vi "TrapezoidalMotionProfile.vi"(6 "Initialize":bool, 7 "dt":dbl=0.02 format="%#_13g", 10 "Time":dbl, 11 "Config":T2={"TargetPos"=10.0, "InitalPos"=0.0, "FinalVel"=0.0, "IntitialVel"=0.0, "MaxVel"=10.0, "MaxAccel"=10.0}) -> (0 "Done":bool, 1 "Acceleration":dbl, 2 "Velocity":dbl, 3 "Distance":dbl)   [LabVIEW 2018]
panel:
  out "AllData":T1
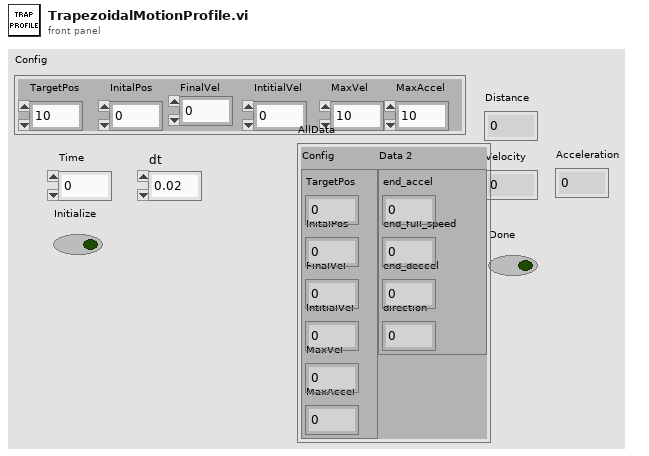
[diagram p1: front panel]
types:
  T1 = cluster{"Config":cluster{"TargetPos":dbl, "InitalPos":dbl, "FinalVel":dbl, "IntitialVel":dbl, "MaxVel":dbl, "MaxAccel":dbl}, "Data 2":cluster{"end_accel":dbl, "end_full_speed":dbl, "end_deccel":dbl, "direction":dbl}}
  T2 = cluster{"TargetPos":dbl, "InitalPos":dbl, "FinalVel":dbl, "IntitialVel":dbl, "MaxVel":dbl, "MaxAccel":dbl}
  T3 = cluster{"end_accel":dbl, "end_full_speed":dbl, "end_deccel":dbl, "direction":dbl}
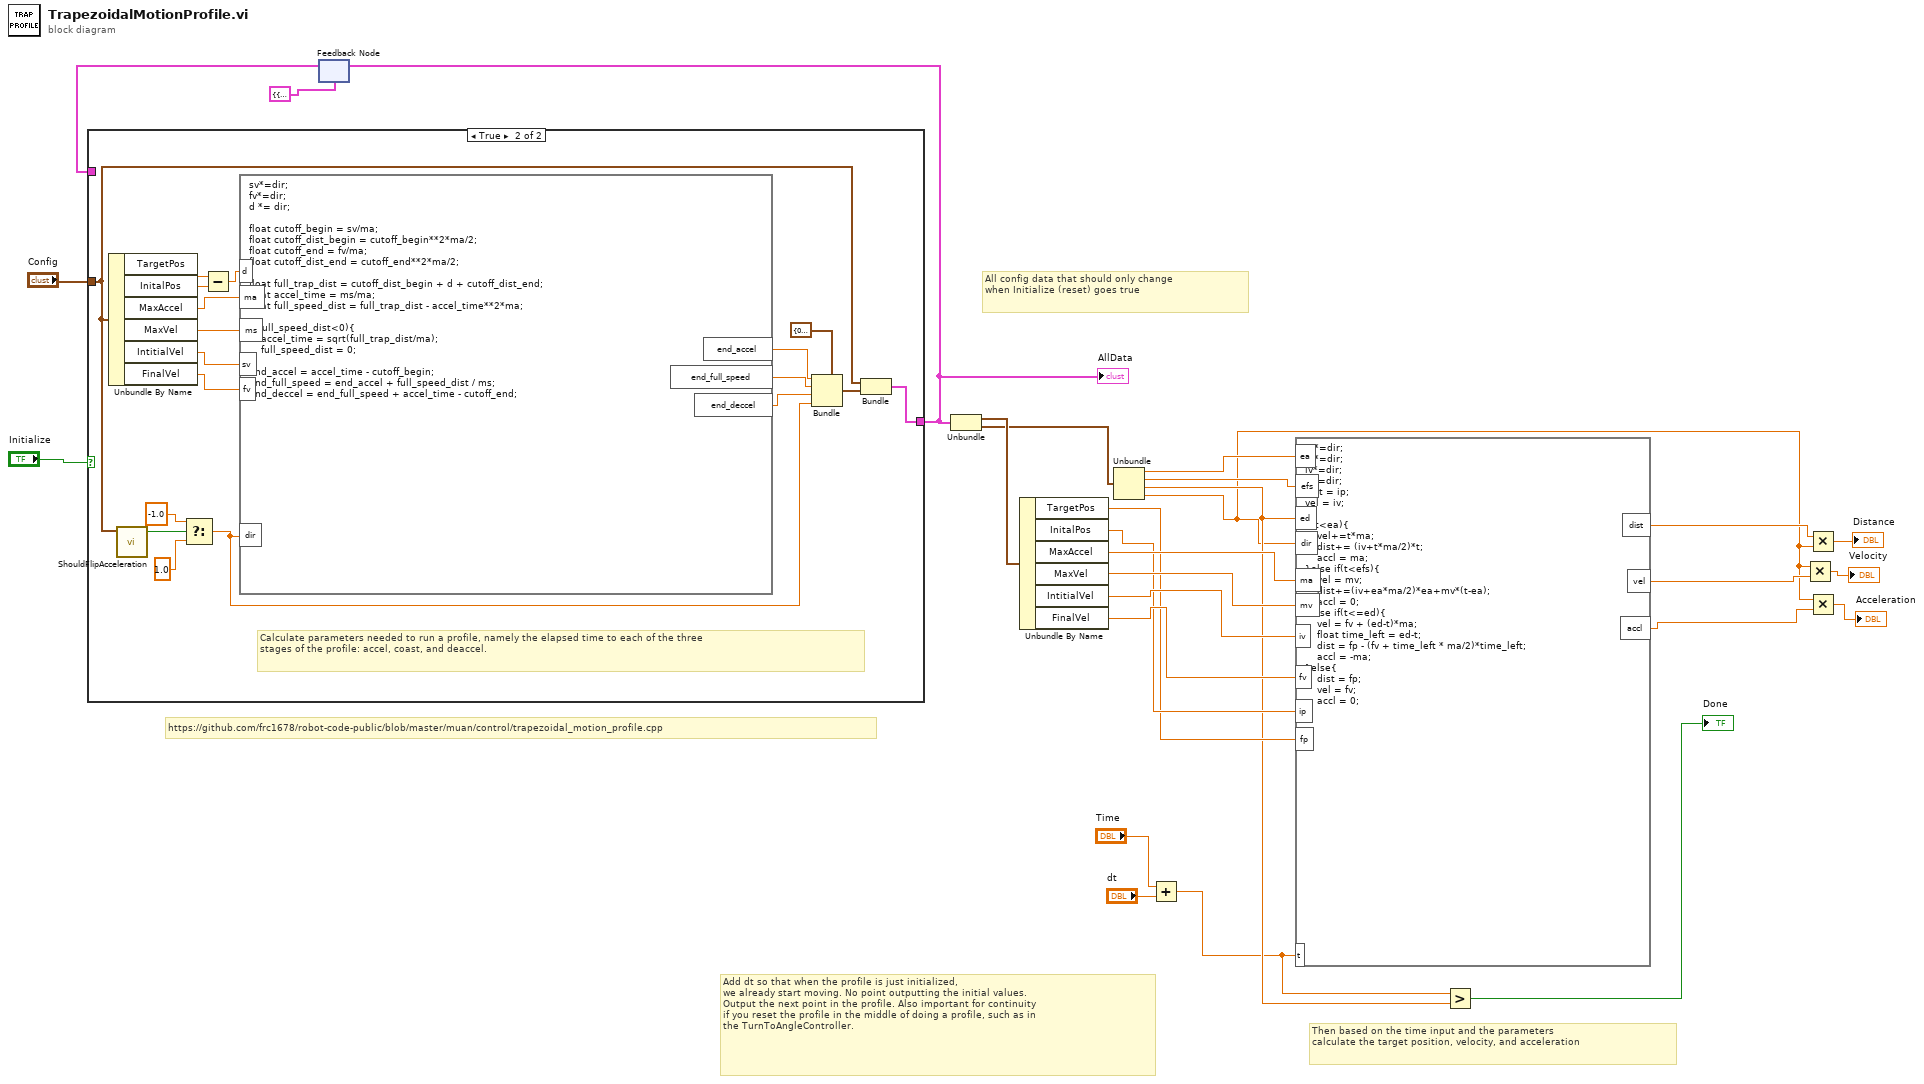
[diagram p0: block diagram]
diagram:
  # "Add dt so that when the profile is just initialized,\nwe already start moving. No point outputting the initial values.\nOutput the next point in the profile. Also important for continuity\nif you reset the profile in the middle of doing a profile, such as in\nthe TurnToAngleController."
  # "Then based on the time input and the parameters\ncalculate the target position, velocity, and acceleration"
  # "All config data that should only change\nwhen Initialize (reset) goes true"
  # "https://github.com/frc1678/robot-code-public/blob/master/muan/control/trapezoidal_motion_profile.cpp"
  n1 = feedback #1(T1 {"Config"={"TargetPos"=10.0, "InitalPos"=0.0, "FinalVel"=0.0, "IntitialVel"=0.0, "MaxVel"=10.0, "MaxAccel"=10.0}, "Data 2"={"end_accel"=0.0, "end_full_speed"=0.0, "end_deccel"=0.0, "direction"=0.0}} ("AllData")) -> (w25:T1)
  n2 = case shown="True" "Initialize" {
    tunnel: "Config" -> [_ w39]
    tunnel: [w28 w29] -> w12
    tunnel: w25 -> [w28 _]
    frame False {
      # "Pass the values through"
    }
    frame True {
      # "Calculate parameters needed to run a profile, namely the elapsed time to each of the three\nstages of the profile: accel, coast, and deaccel."
      n3 = Unbundle By Name(w39) -> ("TargetPos"=w40:dbl, "InitalPos"=w41:dbl, "MaxAccel"=w46:dbl, "MaxVel"=w45:dbl, "IntitialVel"=w43:dbl, "FinalVel"=w42:dbl)
      n4 = call "ShouldFlipAcceleration.vi"("Config"=w39) -> ("Flip?"=w35:bool)  [unwired: 10 in]
      n5 = Select(t=-1.0, s=w35, f=1.0) -> (s? t:f=w30:dbl)
      n6 = Subtract(x=w40, y=w41) -> (x-y=w44:dbl)
      n7 = formula code="sv*=dir;\nfv*=dir;\nd *= dir;\n\nfloat cutoff_begin = sv/ma;\nfloat cutoff_dist_begin = cutoff_begin**2*ma/2;\nfloat cutoff_end = fv/ma;\nfloat cutoff_dist_end = cutoff_end**2*ma/2;\n\nfloat full_trap_dist = cutoff_dist_begin + d + cutoff_dist_end;\nfloat accel_time = ms/ma;\nfloat full_speed_dist = full_trap_dist - accel_time**2*ma;\n\nif(full_speed_dist<0){\n    accel_time = sqrt(full_trap_dist/ma);\n    full_speed_dist = 0;\n}\nend_accel = accel_time - cutoff_begin;\nend_full_speed = end_accel + full_speed_dist / ms;\nend_deccel = end_full_speed + accel_time - cutoff_end;"("ma"=w46, "ms"=w45, "d"=w44, "sv"=w43, "fv"=w42, "dir"=w30) -> ("end_accel"=w37:dbl, "end_full_speed"=w32:dbl, "end_deccel"=w31:dbl)
      n8 = Bundle(cluster=T3 {"end_accel"=0.0, "end_full_speed"=0.0, "end_deccel"=0.0, "direction"=0.0} ("Data 2"), "end_accel"=w37, "end_full_speed"=w32, "end_deccel"=w31, "direction"=w30) -> (w38:T3)
      n9 = Bundle("Config"=w39, "Data 2"=w38) -> (w29:T1)  [unwired: 1 in]
    }
  }
  "AllData" <- w12
  n10 = feedback-in #1(w12) -> ()
  n11 = Unbundle(w12) -> ("Config"=w11:T2, "Data 2"=w10:T3)
  n12 = Unbundle By Name(w11) -> ("TargetPos"=w18:dbl, "InitalPos"=w19:dbl, "MaxAccel"=w23:dbl, "MaxVel"=w22:dbl, "IntitialVel"=w21:dbl, "FinalVel"=w20:dbl)
  n13 = Unbundle(w10) -> ("end_accel"=w17:dbl, "end_full_speed"=w16:dbl, "end_deccel"=w15:dbl, "direction"=w6:dbl)
  n14 = Add(x="Time", y="dt") -> (x+y=w2:dbl)
  n15 = formula code="ip*=dir;\nfp*=dir;\niv*=dir;\nfv*=dir;\ndist = ip;\nvel = iv;\n\nif(t<ea){\n    vel+=t*ma;\n    dist+= (iv+t*ma/2)*t;\n    accl = ma;\n}else if(t<efs){\n    vel = mv;\n    dist+=(iv+ea*ma/2)*ea+mv*(t-ea);\n    accl = 0;\n}else if(t<=ed){\n    vel = fv + (ed-t)*ma;\n    float time_left = ed-t;\n    dist = fp - (fv + time_left * ma/2)*time_left;\n    accl = -ma;\n}else{\n    dist = fp;\n    vel = fv;\n    accl = 0;\n}"("t"=w2, "ea"=w17, "efs"=w16, "ed"=w15, "ma"=w23, "iv"=w21, "mv"=w22, "fv"=w20, "ip"=w19, "fp"=w18, "dir"=w6) -> ("dist"=w14:dbl, "vel"=w13:dbl, "accl"=w5:dbl)
  n16 = Greater?(x=w2, y=w15) -> (0:→"Done":bool)
  n17 = Multiply(x=w6, y=w13) -> (x*y=→"Velocity":dbl)
  n18 = Multiply(x=w14, y=w6) -> (x*y=→"Distance":dbl)
  n19 = Multiply(x=w6, y=w5) -> (x*y=→"Acceleration":dbl)
